vi "HapticSPM_read.vi"() -> ()   [LabVIEW 2021]
uses:
  Program Files/National Instruments/LabVIEW 2022/user.lib/Haptic Prog Interface/Haptic Prog Interface.lvlib
  Program Files/National Instruments/LabVIEW 2022/user.lib/Nanonis Prog Interface V5/Nanonis Prog Interface.lvlib
panel:
  out "Number of Clicks":i8
  in  "Reset":bool
  out "x*y":dbl
  in  "Force Settings":u16(ring) items=["0", "1", "2", "3", "4"]
  in  "Fine":dbl
  in  "Rough":dbl
  out "Reframed Position (m)":cluster{"x (m)":dbl, "y (m)":dbl, "z (m)":dbl} {"z (m)" format="%.1p"; "y (m)" format="%.1p"; "x (m)" format="%.1p"}
  out "Z position (m)":sgl format="%#_6p"
  out "Center coordinates (m)":cluster{"Xc":sgl, "Yc":sgl} {"Yc" format="%.2p"; "Xc" format="%.2p"}
  out "Size (m)":cluster{"Width":sgl, "Height":sgl} {"Height" format="%.2p"; "Width" format="%.2p"}
  out "Angle (deg)":sgl format="%.2f"
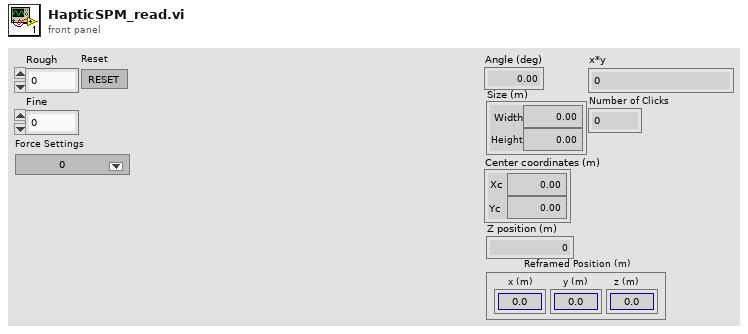
[diagram p1: front panel]
types:
  T1 = cluster{"Center coordinates (m)":cluster{"Xc":sgl, "Yc":sgl}, "Size (m)":cluster{"Width":sgl, "Height":sgl}}
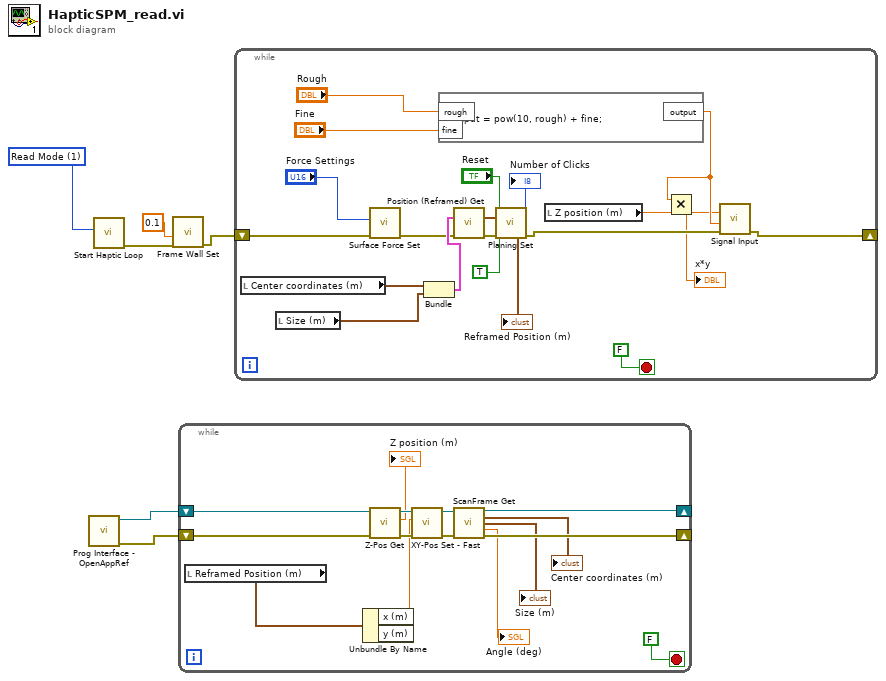
[diagram p0: block diagram]
diagram:
  w6 = u16 1 items=["Custom Mode", "Read Mode", "Write Mode"] ("Mode Selection")
  n1 = call <userlib>:"Prog Interface - OpenAppRef.vi"() -> ("Error out"=w5:errorcluster, "Application reference"=w1:refnum<vi>)  [unwired: 6 in]
  n2 = call "Start Haptic Loop.vi"("Mode Selection"=w6) -> ("error out"=w3:errorcluster)  [unwired: 10 in]
  n3 = call "Frame Wall Set.vi"("error in (no error)"=w3, "Wall Stiffness (N/m)"=0.1) -> ("error out"=w4:errorcluster)  [unwired: 9 in]
  n4 = while {
    shift-right: [w18] -> _
    shift-left: w5 -> [w21]
    shift-right: [w11] -> _
    shift-left: w1 -> [w14]
    stop <- FALSE stop-if-true
    n5 = local read "Reframed Position (m)"() -> (w9:cluster{"x (m)":dbl, "y (m)":dbl, "z (m)":dbl})
    n6 = Unbundle By Name(w9) -> ("x (m)"=w8:dbl, "y (m)"=w7:dbl)
    n7 = call <userlib>:"Z-Pos Get.vi"("error in (no error)"=w21, "Application ref in"=w14) -> ("error out"=w20:errorcluster, "Z position (m)"=→"Z position (m)":sgl, "Application ref out"=w13:refnum<vi>)  [unwired: 7 in]
    n8 = call <userlib>:"XY-Pos Set - Fast.vi"("error in (no error)"=w20, "Y (m)"=w7, "X (m)"=w8, "Application ref in"=w13) -> ("error out"=w19:errorcluster, "Application ref out"=w12:refnum<vi>)  [unwired: 5 in]
    n9 = call <userlib>:"ScanFrame Get.vi"("Application ref in"=w12, "error in (no error)"=w19) -> ("Application ref out"=w11:refnum<vi>, "Center coordinates (m)"=→"Center coordinates (m)":cluster{"Xc":sgl, "Yc":sgl}, "Size (m)"=→"Size (m)":cluster{"Width":sgl, "Height":sgl}, "Angle (deg)"=→"Angle (deg)":sgl, "error out"=w18:errorcluster)  [unwired: 9 in]
  }
  n10 = while {
    shift-right: [w33] -> _
    shift-left: w4 -> [w39]
    stop <- FALSE stop-if-true
    n11 = local read "Center coordinates (m)"() -> (w38:cluster{"Xc":sgl, "Yc":sgl})
    n12 = local read "Size (m)"() -> (w37:cluster{"Width":sgl, "Height":sgl})
    n13 = call "Surface Force Set.vi"("error in (no error)"=w39, "Force Settings"="Force Settings") -> ("error out"=w30:errorcluster)  [unwired: 9 in]
    n14 = Bundle("Center coordinates (m)"=w38, "Size (m)"=w37) -> (w36:T1)  [unwired: 1 in]
    n15 = formula code="output = pow(10, rough) + fine;"("rough"="Rough", "fine"="Fine") -> ("output"=w28:dbl)
    n16 = call "Position (Reframed) Get.vi"("Frame Properties (m)"=w36, "error in (no error)"=w30) -> ("Reframed Position (m)"=→"Reframed Position (m)":cluster{"x (m)":dbl, "y (m)":dbl, "z (m)":dbl}, "error out"=w40:errorcluster)  [unwired: 12 in]
    n17 = call "Planing Set.vi"("error in (no error)"=w40, "Planing"=TRUE, "Reset"="Reset") -> ("error out"=w34:errorcluster, "Number of Clicks"=→"Number of Clicks":i8)  [unwired: 7 in]
    n18 = local read "Z position (m)"() -> (w26:sgl)
    n19 = Multiply(x=w28, y=w26) -> (x*y=→"x*y":dbl)
    n20 = call "Signal Input.vi"("error in (no error)"=w34, "Gain"=w28, "Signal"=w26) -> ("error out"=w33:errorcluster)  [unwired: 8 in]
  }
